vi "TestTemp Slider.vi"() -> ()   [LabVIEW 2017]
panel:
  in  "Temperature Slider":dbl(slide) scale=0.0..10.0
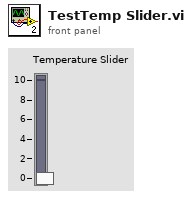
[diagram p1: front panel]
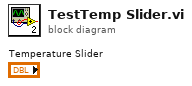
[diagram p0: block diagram]
diagram:
